vi "Extract First Two.vi"(10 "Array":dbl[](array[numeric])) -> (2 "Output Cluster":T1)   [LabVIEW 2017]
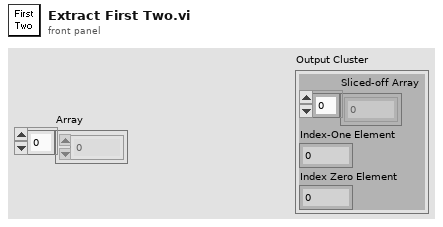
[diagram p1: front panel]
types:
  T1 = cluster{"Sliced-off Array":dbl[], "Index-One Element":dbl, "Index Zero Element":dbl}
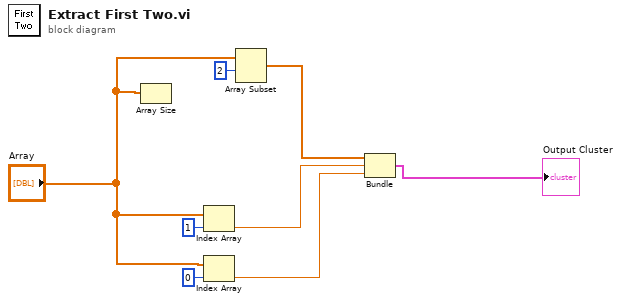
[diagram p0: block diagram]
diagram:
  n1 = Array Size(array="Array") -> ()  [unwired: 1 out]
  n2 = Index Array(array="Array", index=1) -> (element=w3:dbl)
  n3 = Index Array(array="Array", index=0) -> (element=w2:dbl)
  n4 = Array Subset(array="Array", index=2) -> (w4:dbl[])  [unwired: 1 in]
  n5 = Bundle(w4, "Numeric"=w3, "Numeric"=w2) -> (→"Output Cluster":cluster{dbl[], "Numeric":dbl, "Numeric":dbl})  [unwired: 1 in]
